vi "prepareSubpanelMethods.vi"(8 "error in (no error)":errorcluster, 11 "ViewThisComponent in":refnum<class "ViewThisComponent.lvclass">) -> (0 "error out":errorcluster, 3 "ViewThisComponent out":refnum<class "ViewThisComponent.lvclass">)   [LabVIEW 2015, in "ViewThisComponent.lvclass"]
doc: "Sets the value of the \"view\" control on each of the views in the subpanel to a View object equipped with the valid viewUserEvent."
uses:
  ViewThisComponent.lvclass
  ComponentTemplateCore/ComponentModel/ComponentModel/View/View.lvclass/View.ctl
  ViewThisComponent.lvclass/ViewThisComponent.ctl
  ComponentTemplateCore/ComponentModel/ComponentModel/View/View.lvclass
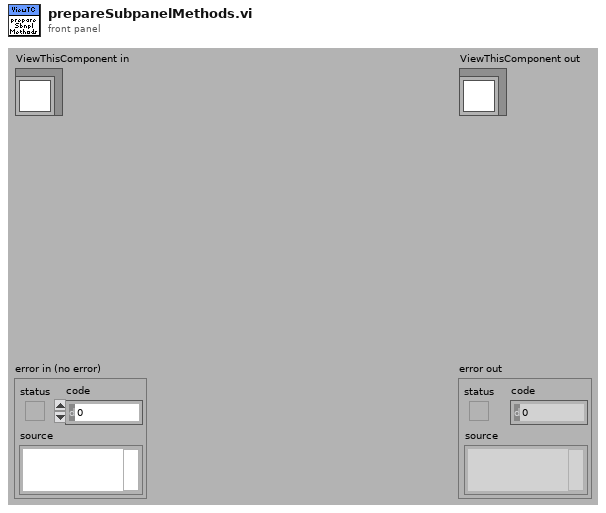
[diagram p1: front panel]
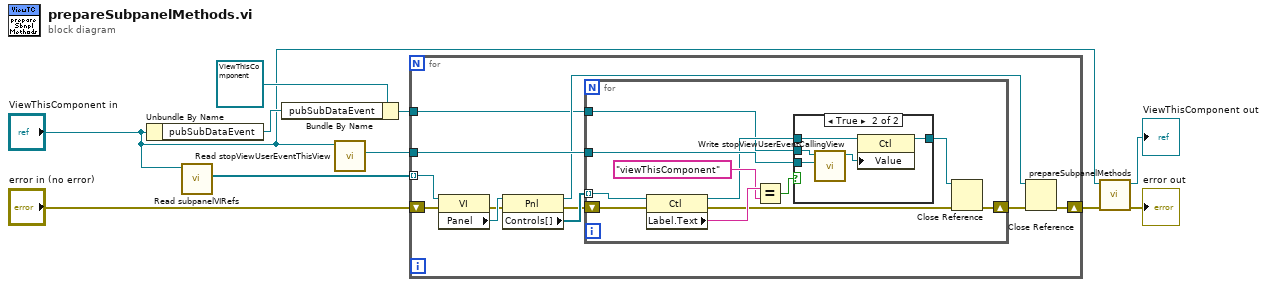
[diagram p0: block diagram]
diagram:
  n1 = Unbundle By Name("ViewThisComponent in") -> ("pubSubDataEvent"=w5:refnum<class "PubSubDataEvent.lvclass">)
  n2 = call "Read subpanelVIRefs.vi"("View in"="ViewThisComponent in") -> ("subpanelVIRefs"=w8:refnum<vi>[])  [unwired: 9 in, 1 out]
  n3 = Bundle By Name(cluster=refnum<class "ViewThisComponent.lvclass"> refnum ("ViewThisComponent.lvclass"), "pubSubDataEvent"=w5) -> (w6:refnum<class "ViewThisComponent.lvclass">)
  n4 = call "Read stopViewUserEventThisView.vi"("View in"="ViewThisComponent in") -> ("stopViewUserEventThisView"=w9:refnum<user-event>)  [unwired: 9 in, 1 out]
  n5 = for {
    tunnel: w8 -> [w21] mode=indexing
    tunnel: w9 -> [w18]
    shift-right: [w12] -> w3
    shift-left: "error in (no error)" -> [w16]
    tunnel: w6 -> [w11]
    n6 = property class="VI"(reference=w21, error in=w16) -> (error out=w15:errorcluster, "Panel"=w20:refnum<vi>)  [unwired: 1 out]
    n7 = property class="Pnl"(reference=w20, error in=w15) -> (reference out=w17:refnum<vi>, error out=w14:errorcluster, "Controls[]"=w19:refnum<vi>[])
    n8 = for {
      tunnel: w19 -> [w32] mode=indexing
      tunnel: w18 -> [w28]
      shift-right: [w23] -> w13
      shift-left: w14 -> [w25]
      tunnel: w11 -> [w22]
      n9 = property class="Ctl"(reference=w32, error in=w25) -> (reference out=w26:refnum<vi>, error out=w24:errorcluster, "Label.Text"=w31:string)
      n10 = Equal?(x=w31, y="viewThisComponent") -> (x = y?=w29:bool)
      n11 = case shown="True" w29 {
        tunnel: w28 -> [_ w36]
        tunnel: [w33 w37] -> w27
        tunnel: w26 -> [w33 w38]
        tunnel: w22 -> [_ w35]
        frame False {
        }
        frame True {
          n12 = call "Write stopViewUserEventCallingView.vi"("stopViewUserEventCallingView"=w36, "View in"=w35) -> ("View out"=w34:refnum<class "ViewThisComponent.lvclass">)  [unwired: 9 in]
          n13 = property class="Ctl"(reference=w38, "Value"=w34) -> (reference out=w37:refnum<vi>)  [unwired: 1 in, 1 out]
        }
      }
      n14 = Close Reference(reference=w27, error in (no error)=w24) -> (error out=w23:errorcluster)
    }
    n15 = Close Reference(reference=w17, error in (no error)=w13) -> (error out=w12:errorcluster)
  }
  n16 = call-parent "prepareSubpanelMethods.vi"("error in (no error)"=w3, "View in"="ViewThisComponent in") -> ("error out"=→"error out":errorcluster, "View out"=→"ViewThisComponent out":refnum<class "ViewThisComponent.lvclass">)  [unwired: 8 in]
